vi "AMC e.bloxx Example - Get All Module Informations.vi"() -> ()   [LabVIEW 2013]
doc: "<B>AMC - Analytik & Messtechnik GmbH Chemnitz</B>\n\nLabVIEW Drivers for e.bloxx series from Gantner Instruments\n\nThis example demonstrates the usage of the e.bloxx VIs. You must select your serial settings according to the e.bloxx configuration set via ICP software. Then choose your designated module by Module Address. All informations about the module should appear on the front panel."
uses:
  AMC e.bloxx Module Error.ctl
  AMC e.bloxx Variable Information.ctl
  AMC e.bloxx Variable Type.ctl
  AMC e.bloxx Data Format.ctl
  AMC e.bloxx Host Input.ctl
panel:
  out "error out":errorcluster
  out "Variable Informations":T1[](array[typedef]) {"Host Input" items=["Not Possible"=48, "Possible"=49]; "Data Format" items=["No Format"=48, "Boolean"=49, "Integer"=52, "Long"=54, "Real"=56, "Set 8"=57]; "Variable Type" items=["Empty"=48, "Analog Input"=49, "Arithmetic"=50, "Digital Output"=51, "Digital Input"=52, "Setpoint"=53, "Alarm"=54, "Controller"=57]}
  out "Location":string
  out "Serial Number":i32
  out "Any Errors?":bool
  out "Module Errors":T5[](array[typedef]) items=["EEPROM Error", "FLASH Error", "ADC Error", "Configuration Error"]
  out "Channel Status":i32
  out "Software Revision":string
  out "Model Name":string
  out "Vendor Name":string
  out "Hardware Revision":string
  in  "Module Address":i32=2
  in  "Parity":enum16{"None", "Odd", "Even", "Mark", "Space"}(ring)=enum."Even"
  in  "Baudrate":u32=115200
  in  "VISA Resource Name":refnum<visa-resource-name>="COM2"
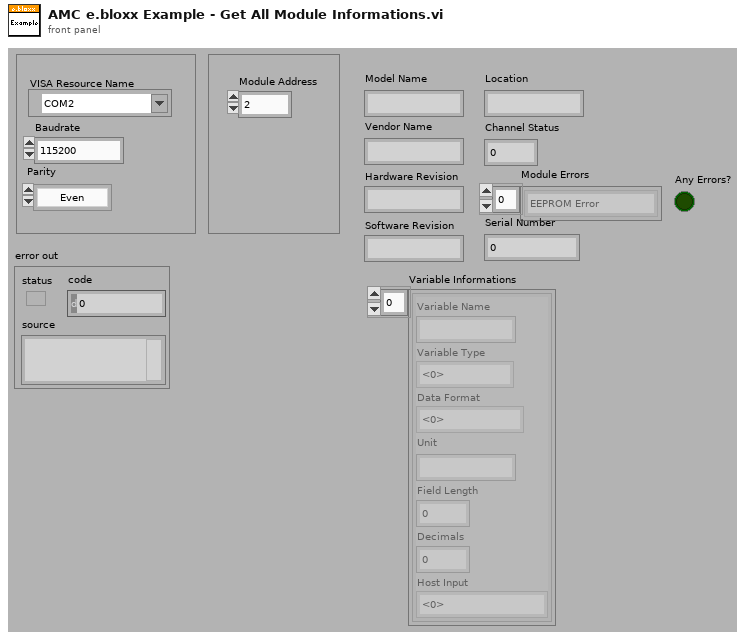
[diagram p1: front panel]
types:
  T1 = typedef "AMC e.bloxx Variable Information.ctl" = cluster{"Variable Name":string, "Variable Type":T2, "Data Format":T3, "Unit":string, "Field Length":u8, "Decimals":u8, "Host Input":T4}
  T2 = typedef "AMC e.bloxx Variable Type.ctl" = u8
  T3 = typedef "AMC e.bloxx Data Format.ctl" = u8
  T4 = typedef "AMC e.bloxx Host Input.ctl" = u8
  T5 = typedef "AMC e.bloxx Module Error.ctl" = i32
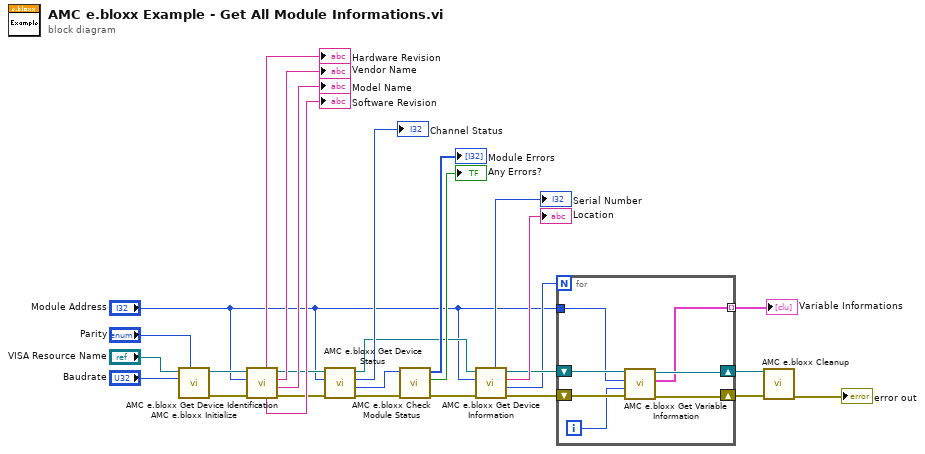
[diagram p0: block diagram]
diagram:
  n1 = call "AMC e.bloxx Initialize.vi"("parity (0:none)"="Parity", "baud rate (9600)"="Baudrate", "VISA resource name"="VISA Resource Name") -> ("error out"=w24:errorcluster, "VISA resource name out"=w25:refnum<visa-resource-name>)  [unwired: 7 in]
  n2 = call "AMC e.bloxx Get Device Identification.vi"("error in (no error)"=w24, "Module Address"="Module Address", "VISA Resource Name"=w25) -> ("error out"=w18:errorcluster, "Model Name"=→"Model Name":string, "Vendor Name"=→"Vendor Name":string, "VISA Resource Name out"=w19:refnum<visa-resource-name>, "Software Revision"=→"Software Revision":string, "Hardware Revision"=→"Hardware Revision":string)  [unwired: 3 in]
  n3 = call "AMC e.bloxx Get Device Status.vi"("error in (no error)"=w18, "Module Address"="Module Address", "VISA Resource Name"=w19) -> ("error out"=w15:errorcluster, "Module Status"=w16:i32, "Channel Status"=→"Channel Status":i32, "VISA Resource Name out"=w11:refnum<visa-resource-name>)  [unwired: 5 in]
  n4 = call "AMC e.bloxx Check Module Status.vi"("error in (no error)"=w15, "Module Status"=w16) -> ("error out"=w12:errorcluster, "Any Errors?"=→"Any Errors?":bool, "Module Errors"=→"Module Errors":T5[])  [unwired: 7 in]
  n5 = call "AMC e.bloxx Get Device Information.vi"("error in (no error)"=w12, "Module Address"="Module Address", "VISA Resource Name"=w11) -> ("error out"=w7:errorcluster, "Channel Count"=w6:i32, "Location"=→"Location":string, "VISA Resource Name out"=w8:refnum<visa-resource-name>, "Serial Number"=→"Serial Number":i32)  [unwired: 4 in]
  n6 = for {
    N: w6 -> [_]
    shift-right: [w30] -> w3
    shift-left: w8 -> [w35]
    shift-right: [w31] -> w2
    shift-left: w7 -> [w34]
    tunnel: "Module Address" -> [w33]
    tunnel: [w29] -> w4 mode=indexing
    i -> [w32]
    n7 = call "AMC e.bloxx Get Variable Information.vi"("error in (no error)"=w34, "Variable"=w32, "Module Address"=w33, "VISA Resource Name"=w35) -> ("error out"=w31:errorcluster, "Variable Information"=w29:T1, "VISA Resource Name out"=w30:refnum<visa-resource-name>)  [unwired: 5 in]
  }
  "Variable Informations" <- w4
  n8 = call "AMC e.bloxx Cleanup.vi"("error in (no error)"=w2, "VISA resource name"=w3) -> ("error out"=→"error out":errorcluster)  [unwired: 9 in]
